vi "TCTest.vi"() -> ()   [LabVIEW 2022 SP3]
doc: "Cont(inuous) Acq(uire) & Chart (immediate) demonstrates the software timed, non-buffered technique of data acquisition. Timing functions control the timing of the loop and in each loop AI Single Scan is called to read an immediate scan of the channels listed. Each scan is plotted on the chart after it is read. This example uses the lower level intermediate VIs: AI Config and AI Single Scan.\n\nSee Cont Acq&Chart (easy immed) for a functionally identical but simpler version using a single higher level intermediate VI. This example is also similar to the Cont Acq&Chart (hw timed) and (buffered) examples.\n\nA common reason to use untimed, immediate acquisition is that some kind of processing needs to be done for each data point. You will probably want to add more functions to the diagram to customize this VI for your application. The acquisition rate you can achieve depends on how much processing and display the VI must do. This VI calls a subVI named My Single-Scan Processing. Add whatever processing you need to this subVI, or replace it with one of your own. The data processing subVI also demonstrates how to use error clusters in your own subVIs, so they can be included in the error data flow chain.\n\nBefore running this VI, set the values of the controls on the front panel. Select Show Help Window from the Help menu to see a description of each control. If the values you select for all the controls are values you will usually use, select Make Current Values Default from the Operate menu and save the VI. Or, you may save individual control's default values by popping up on the control, selecting Data Operations, then selecting Make Current Value Default, and saving the VI."
uses:
  AI Single Scan (scaled array).vi
panel:
  out "Celsius":dbl format="%.2f"
  in  "Happy Number":dbl=295.0 format="%.2f"
  in  "channels (0)":tag[](array[tag])=["ai5 - Sample Temperature CJC", "ai4 - Sample Temperature", "K Thermocouple"]
  out "Actual loop rate":sgl=3.0030031 format="%.2f"
  in  "input limits":cluster{"high limit":sgl, "low limit":sgl}[](array[cluster]) {"low limit" format="%.2f"; "high limit" format="%.2f"}
  in  "interchannel delay\nin secs ( -1: hw default)":sgl=-1.0 max=0.01 format="%.2p"
  in  "scan rate\n(3 scans/sec)":sgl=25.0 min=0.01 max=1000 format="%.2f"
  out "transposed waveform chart":sgl[][](graph)=[[297.16638, 295.98007, 293.51553, 295.0]]
  in  "stop":bool
  in  "device (1)":i16=1
  # "For instructions select File >> VI Properties >> Documentation"
  # "hardware settings"
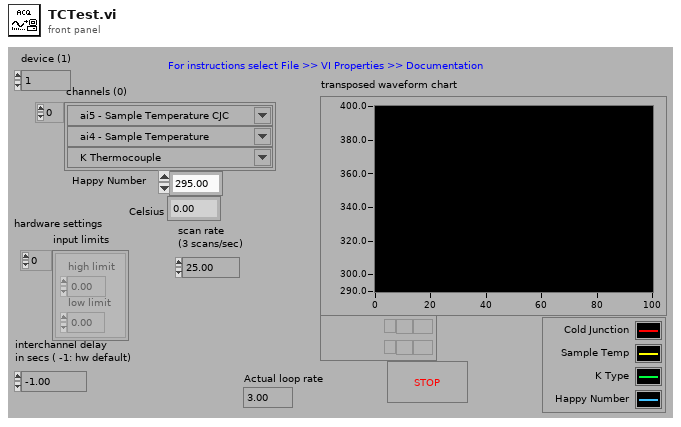
[diagram p1: front panel]
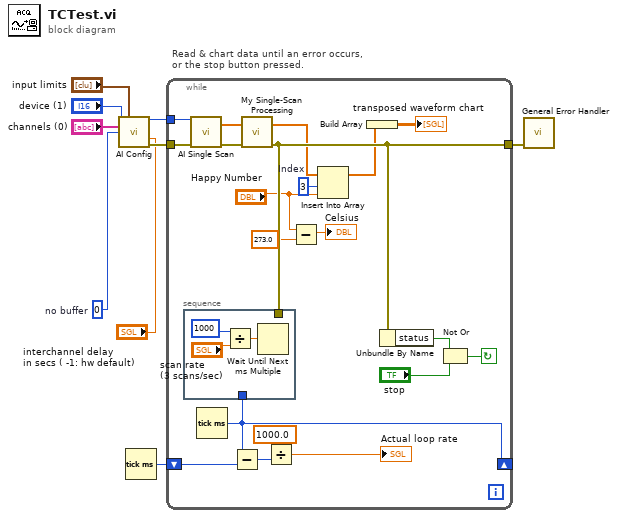
[diagram p0: block diagram]
diagram:
  w8 = 0  # no buffer
  n1 = call "AI Config.vi"("device (1)"="device (1)", "input limits (no change)"="input limits", "channels (0)"="channels (0)", "buffer size (1000 scans)"=w8, "interchannel delay (secs) (board default)"="interchannel delay\nin secs ( -1: hw default)") -> ("taskID"=w7:u32, "error out"=w6:errorcluster)  [unwired: 8 in, 1 out]
  n2 = Tick Count (ms)() -> (millisecond timer value=w2:u32)
  n3 = while "Read & chart data until an error occurs,\nor the stop button pressed." {
    tunnel: w7 -> [w28]
    tunnel: w6 -> [w27]
    tunnel: [w17] -> w4
    shift-right: [w16] -> _
    shift-left: w2 -> [w21]
    stop <- w29 continue-if-true
    w15 = 3  # Index
    n4 = call-poly "AI Single Scan.vi"("taskID in"=w28, "error in (no error)"=w27) -> ("scaled data"=w23:sgl[], "error out"=w22:errorcluster)  [unwired: 9 in, 3 out]
    n5 = Tick Count (ms)() -> (millisecond timer value=w16:u32)
    n6 = Subtract(x=w16, y=w21) -> (x-y=w20:u32)
    n7 = call "My Single-Scan Processing.vi"("error in (no error)"=w22, "voltage data"=w23) -> ("error out"=w17:errorcluster, "processed data"=w14:sgl[])  [unwired: 4 in]
    n8 = stacked-sequence {
      tunnel: w17 -> [_]
      tunnel: w16 -> [_]
      frame #0 {
        n9 = Divide(x=1000, y="scan rate\n(3 scans/sec)") -> (x/y=w32:sgl)
        n10 = Wait Until Next ms Multiple(millisecond multiple=w32) -> ()  [unwired: 1 out]
      }
    }
    n11 = Divide(x=sgl 1000.0, y=w20) -> (x/y=→"Actual loop rate":sgl)
    n12 = Subtract(x="Happy Number", y=273.0) -> (x-y=→"Celsius":dbl)
    n13 = Insert Into Array(array=w14, index=w15, new element="Happy Number") -> (w13:sgl[])
    n14 = Build Array(w13) -> (→"transposed waveform chart":sgl[][])
    n15 = Unbundle By Name(w17) -> ("status"=w24:bool)
    n16 = Not Or(1:"stop", 2:w24) -> (0:w29:bool)
  }
  n17 = call <vilib>:"General Error Handler.vi"("error in (no error)"=w4) -> ()  [unwired: 10 in, 5 out]
